vi "getCellStyle.vi"(8 "error in (no error)":errorcluster, 10 "Style":refnum<class "Style.lvclass">, 11 "MS-Excel in":refnum<class "MS-Excel.lvclass">) -> (0 "error out":errorcluster, 2 "Cell Style":refnum<k24>, 3 "MS-Excel out":refnum<class "MS-Excel.lvclass">)   [LabVIEW 2017, in "LabVIEW NPOI.lvlib" / "MS-Excel.lvclass"]
uses:
  MS-Excel.lvclass
  Styles/Style/Style.lvclass
  D:/Benjamin/Documents/Perso/Code/WC/LabVIEW_NPOI/lib/NPOI 2.1.1/NPOI.dll
  lib/NPOI 2.1.1/NPOI.dll
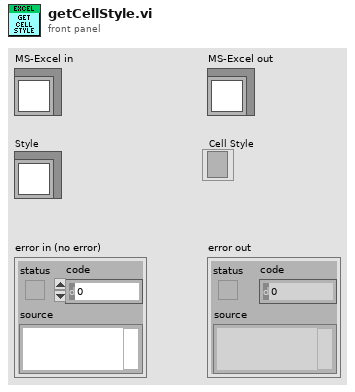
[diagram p1: front panel]
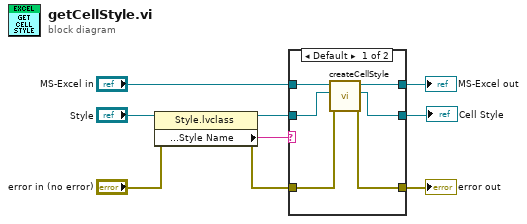
[diagram p0: block diagram]
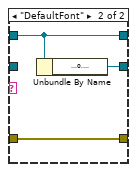
[diagram p2: hidden frame]
diagram:
  n1 = property class="Style.lvclass"(reference="Style", error in="error in (no error)") -> (reference out=w2:refnum<class "Style.lvclass">, error out=w4:errorcluster, "Public VIs:Properties:Style Name"=w7:string)
  n2 = case shown="Default" w7 {
    tunnel: "MS-Excel in" -> [w15 w17]
    tunnel: [w14 w17] -> w5
    tunnel: w4 -> [w12 w18]
    tunnel: [w11 w18] -> w3
    tunnel: w2 -> [w13 _]
    tunnel: [w10 w16] -> w1
    frame Default {
      n3 = call-dynamic "createCellStyle.vi"("error in (no error)"=w12, "Style"=w13, "MS-Excel in"=w15) -> ("error out"=w11:errorcluster, "Cell Style"=w10:refnum<k24>, "MS-Excel out"=w14:refnum<class "MS-Excel.lvclass">)  [unwired: 6 in]
    }
    frame "DefaultFont" {
      n4 = Unbundle By Name(w17) -> ("Cell Style"=w16:refnum<k24>)
    }
  }
  "error out" <- w3
  "MS-Excel out" <- w5
  "Cell Style" <- w1
